vi "Handle Command.vi"(8 "error in (no error)":errorcluster, 9 "Value":bool, 11 "PulsedValve in":refnum<class "PulsedControl.lvclass">) -> (0 "error out":errorcluster, 3 "PulsedValve out":refnum<class "PulsedControl.lvclass">)   [LabVIEW 2020, in "VolatusControl.lvlib" / "PulsedControl.lvclass"]
uses:
  PulsedControl.lvclass
  State.ctl
  PulsedControl.lvclass/PulsedControl.ctl
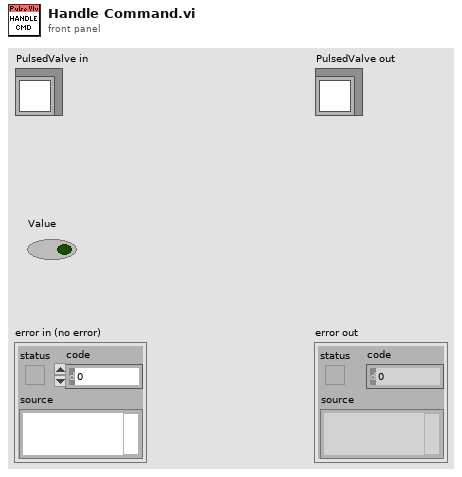
[diagram p1: front panel]
types:
  T1 = typedef "VolatusControl.lvlib/PulsedControl.lvclass/State.ctl" = enum16{"Idle", "Start", "On", "Off"}
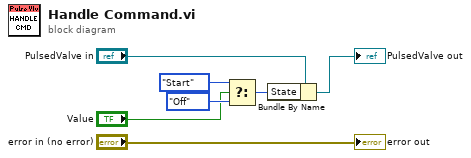
[diagram p0: block diagram]
diagram:
  n1 = Select(t=State."Start" ("State"), s="Value", f=State."Off" ("State")) -> (s? t:f=w1:T1)
  n2 = Bundle By Name(cluster="PulsedValve in", "State"=w1) -> (→"PulsedValve out":refnum<class "PulsedControl.lvclass">)
  "error out" <- "error in (no error)"
